vi "Send Set Analog Read Period.vi"(7 "Message Priority (Normal)":T1=enum."Normal", 8 "error in (no error)":errorcluster, 10 "Loop Period in ms (10)":u32, 11 "Message Enqueuer":refnum<class "Message Enqueuer.lvclass">) -> (0 "error out":errorcluster, 3 "Message Enqueuer out":refnum<class "Message Enqueuer.lvclass">)   [LabVIEW 2024, in "DAQmx Actor.lvlib" / "Set Analog Read Period Msg.lvclass"]
doc: "This VI sends the message to an actor."
uses:
  Set Analog Read Period Msg.lvclass
  <vilib>/ActorFramework/Message Enqueuer/Message Enqueuer.lvclass
  <vilib>/ActorFramework/Message Enqueuer/Message Priority.ctl
  C:/Program Files (x86)/National Instruments/LabVIEW 2024/vi.lib/ActorFramework/Message/Message.lvclass
  Set Analog Read Period Msg.lvclass/Set Analog Read Period Msg.ctl
  <vilib>/ActorFramework/Message Enqueuer/Message Enqueuer.lvclass/Message Enqueuer.ctl
  <vilib>/ActorFramework/Message Priority Queue/Priority Enqueue.vi
  C:/Users/uspoaotto/OneDrive - Oregon Tool/Desktop/working copies/DAQmxActor/src/DAQmx Actor/Analog Reader Messages/Set Analog Read Period Msg/Set Analog Read Period Msg.lvclass
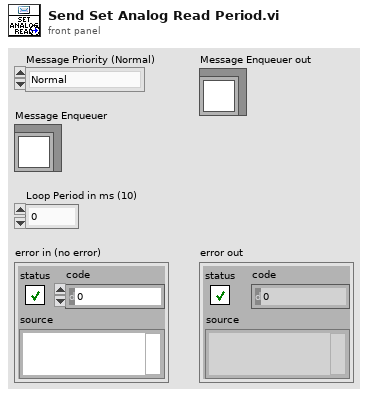
[diagram p1: front panel]
types:
  T1 = typedef "Actor Framework.lvlib/Message Enqueuer.lvclass/Message Priority.ctl" = enum16{"Low", "Normal", "High"}
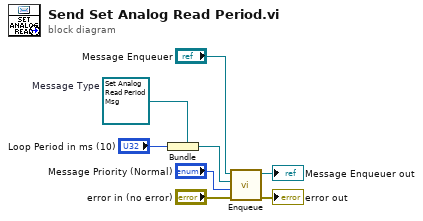
[diagram p0: block diagram]
diagram:
  w5 = refnum<class "Set Analog Read Period Msg.lvclass"> refnum  # Message Type
  n1 = Bundle(cluster=w5, "Loop Period in ms (10)") -> (w4:refnum<class "Set Analog Read Period Msg.lvclass">)
  n2 = call <vilib>:"Enqueue.vi"("error in (no error)"="error in (no error)", "Message Priority (Normal)"="Message Priority (Normal)", "Message"=w4, "Message Enqueuer in"="Message Enqueuer") -> ("error out"=→"error out":errorcluster, "Message Enqueuer in"=→"Message Enqueuer out":refnum<class "Message Enqueuer.lvclass">)  [unwired: 6 in]
